vi "storageLow.vi"(8 "error in (no error)":errorcluster, 11 "reference in":refnum<class "Project Panels.lvclass">=refnum) -> (0 "error out":errorcluster={"status"=TRUE, "code"=1556, "source"="In Place Element Structure in Project Panels.lvclass:items.vi"}, 2 "saved?":bool, 3 "reference out":refnum<class "Project Panels.lvclass">)   [LabVIEW 2016, in "Project Panels.lvclass"]
uses:
  Project Panels.lvclass
  SYS/Items Controller_llb/storageSheets.ctl
  stateItem.ctl
  <vilib>/Utility/miscctls.llb/LVRowAndColumnUnsignedTypeDef.ctl
  <vilib>/Utility/miscctls.llb/LVRowAndColumnTypeDef.ctl
  SYS/Items Controller_llb/Items Controller.lvclass
  SYS/File Controller_llb/File Controller.lvclass
panel:
  out "title":string="Cosmed Asia Pacific - Storage"
  in  "tables":enum32{"Check IN", "Check OUT", "Storage"}(tab)
  in  "checkIN":string[][](table)
  in  "checkOUT":string[][](table)
  in  "Storage":string[][](table)
  in  "uploadFile":bool
  in  "Add Check OUT":bool
  in  "Add Check IN":bool
  out "Number of Items:":i32
  out "index":i32
  in  "back":bool
  in  "next":bool
  out "storageSheets":T1
  in  "Search Item":bool
  in  "Save":bool
  out "Item Selected (S/N or P/N):":string
  out "statuBar":string="Stoped for an Error"
  in  "Stop Button":bool
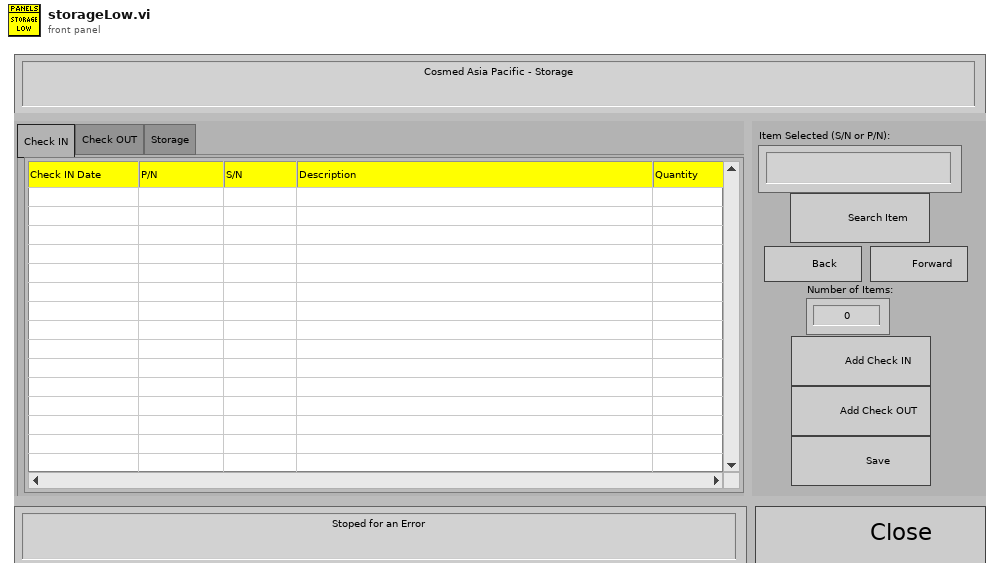
[diagram p1: front panel]
types:
  T1 = typedef "Items Controller.lvclass/storageSheets.ctl" = enum16{"check-in", "check-out", "storage"}
  T2 = typedef "Project Panels.lvclass/stateItem.ctl" = enum16{"initiate", "waitEvent", "save", "search", "UploadFile", "nextItems", "stop"}
  T3 = typedef "LVRowAndColumnUnsignedTypeDef.ctl" = cluster{"Row":u32, "Column":u32}
  T4 = enum8{"Enabled", "Disabled", "Disabled and Grayed Out"}
  T5 = cluster{"checkIN":string[][], "checkOUT":string[][], "storage":string[][]}
  T6 = typedef "LVRowAndColumnTypeDef.ctl" = cluster{"Row":i32, "Column":i32}
  T7 = typedef "Project Panels.lvclass/ObjectAttributesRef.ctl" = refnum<data-value>
  T8 = typedef "Project Panels.lvclass/ObjectAttributes.ctl" = cluster{"MyAttribute":dbl, "device_controller_ref":refnum<class "Devices Controller.lvclass">, "file_controller_ref":refnum<class "File Controller.lvclass">, "item_controller_ref":refnum<class "Items Controller.lvclass">, "item_tables":cluster{"checkIN":string[][], "checkOUT":string[][], "storage":string[][]}, "quickbook_table":cluster{"notes":string[][]}, "notification_controller_ref":refnum<class "Notification Controller.lvclass">, "partstracking_controller_ref":refnum<class "PartsTracking Controller.lvclass">, "product_tables":cluster{"k4b2":string[][], "fitmate":string[][], "RMR":string[][], "CPET":string[][], "BP":string[][], "PP":string[][], "k5":string[][], "bb-pft":string[][]}, "rowsColour":u32[], "low_resolution?":bool, "run_python?":bool}
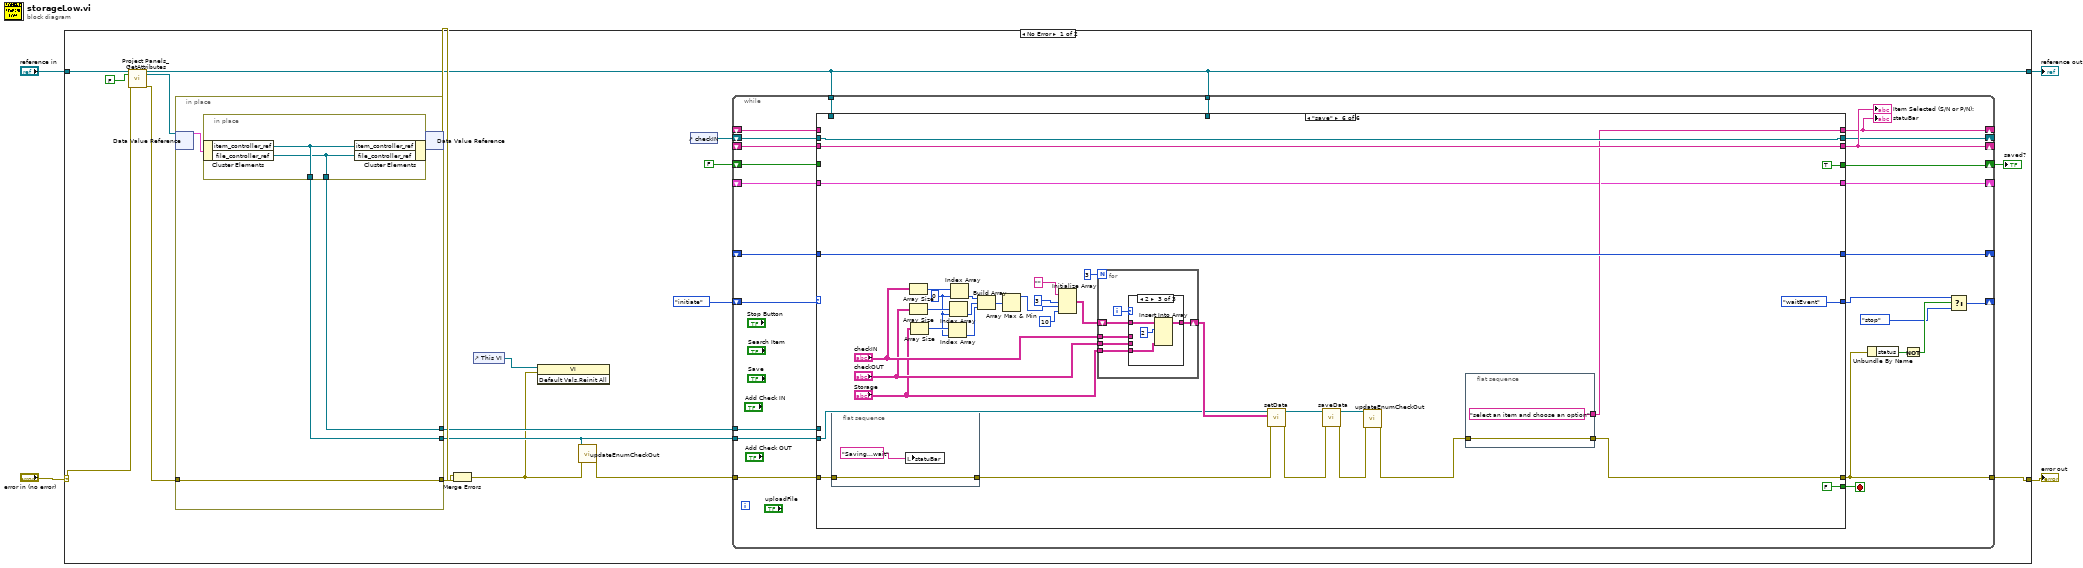
[diagram p0: block diagram]
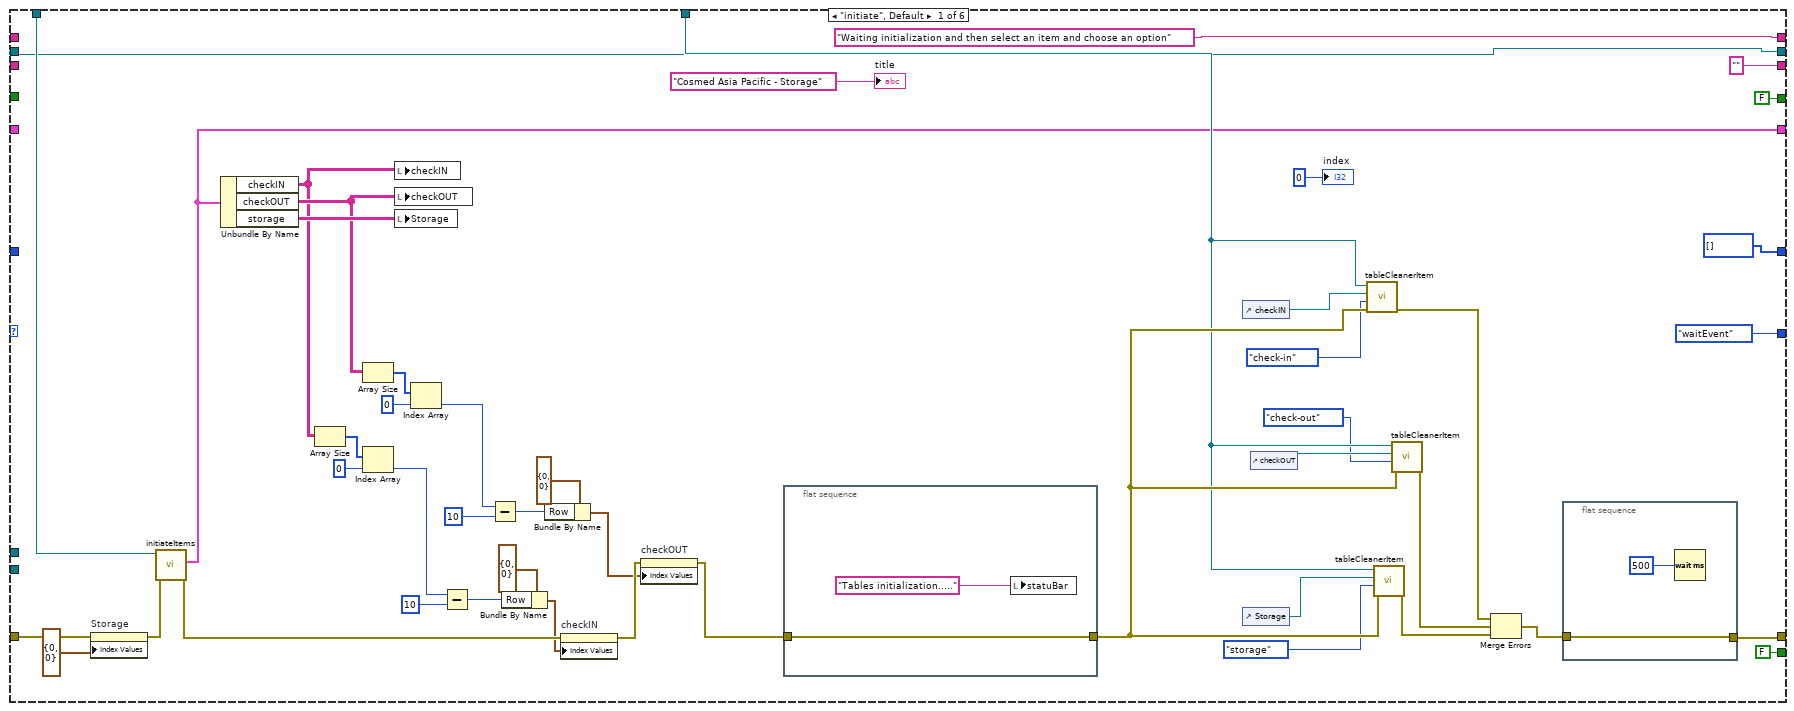
[diagram p2: hidden frame]
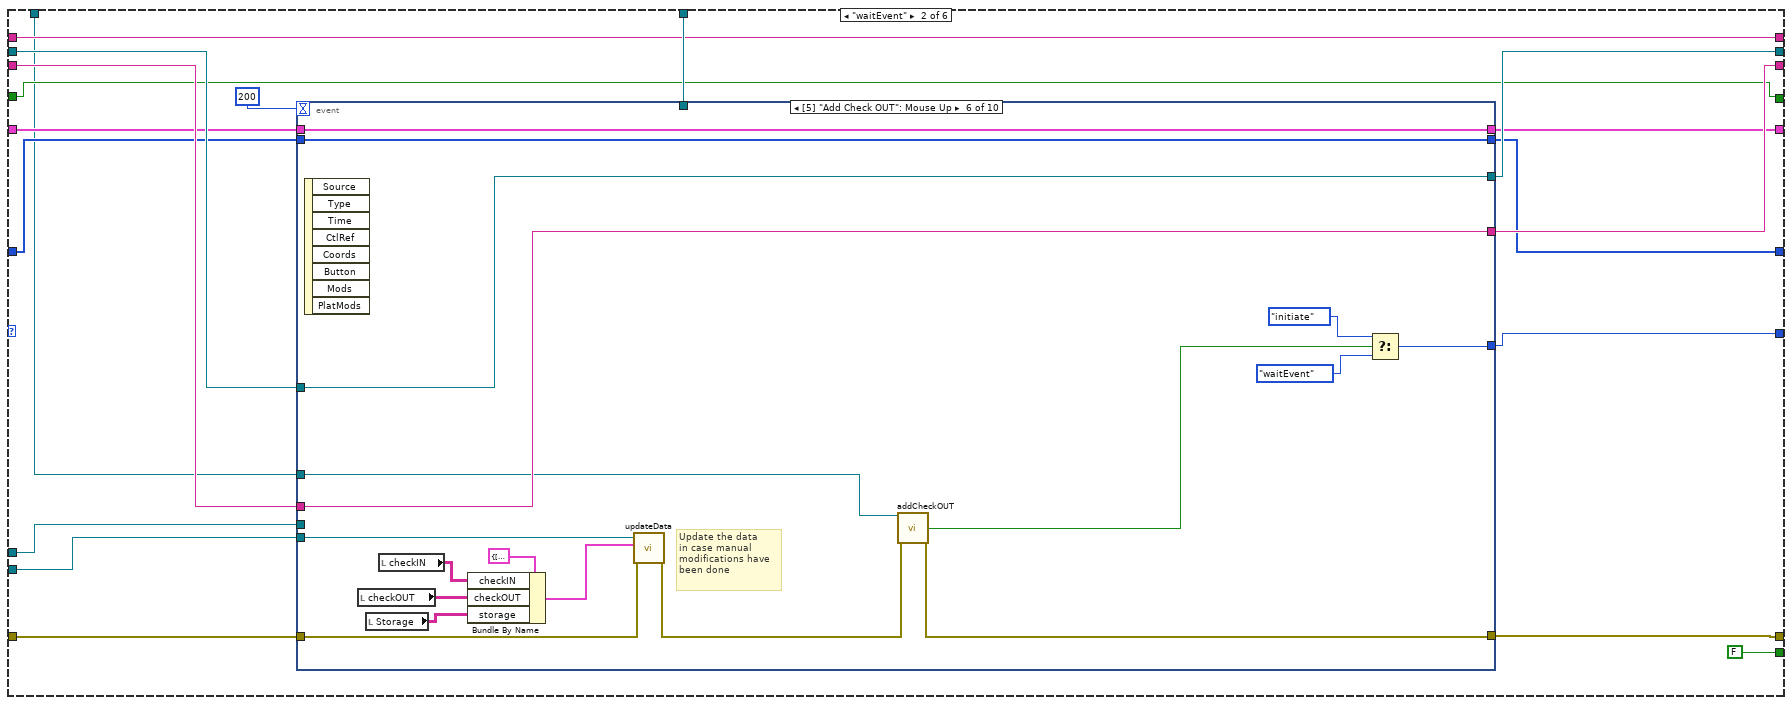
[diagram p3: hidden frame]
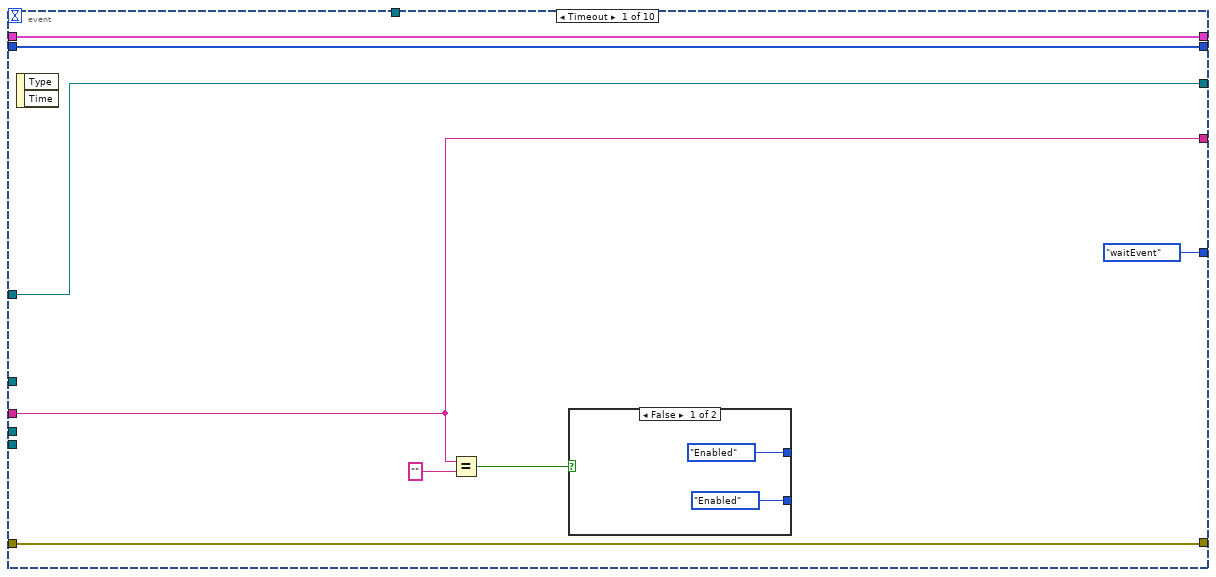
[diagram p4: hidden frame]
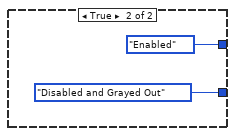
[diagram p5: hidden frame]
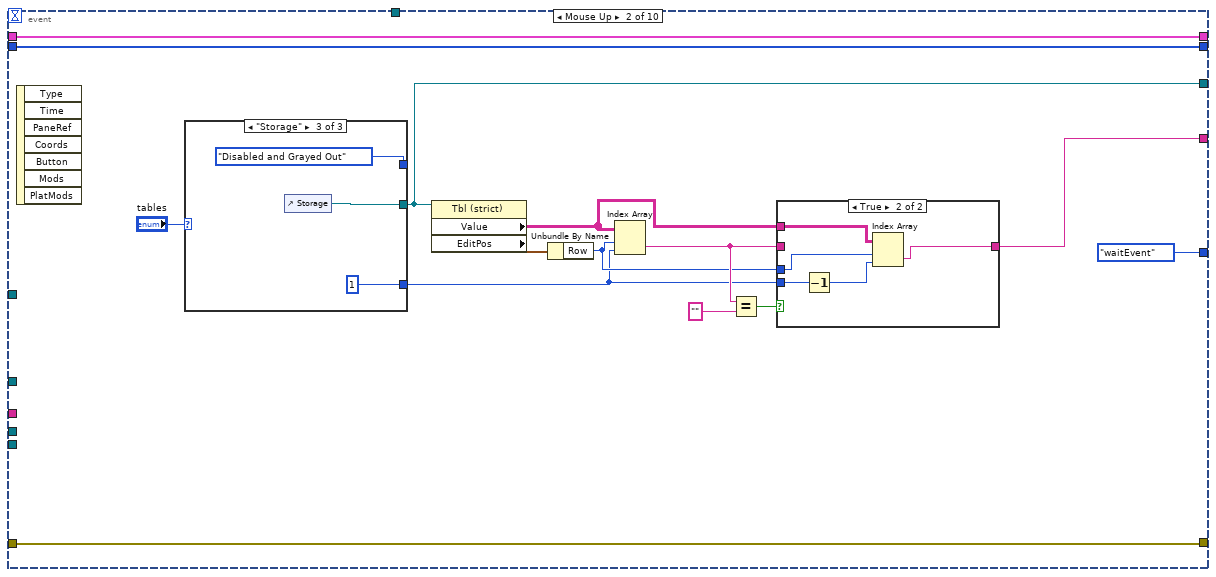
[diagram p6: hidden frame]
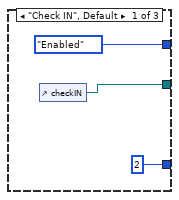
[diagram p8: hidden frame]
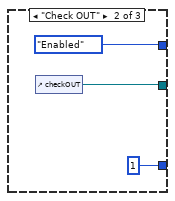
[diagram p9: hidden frame]
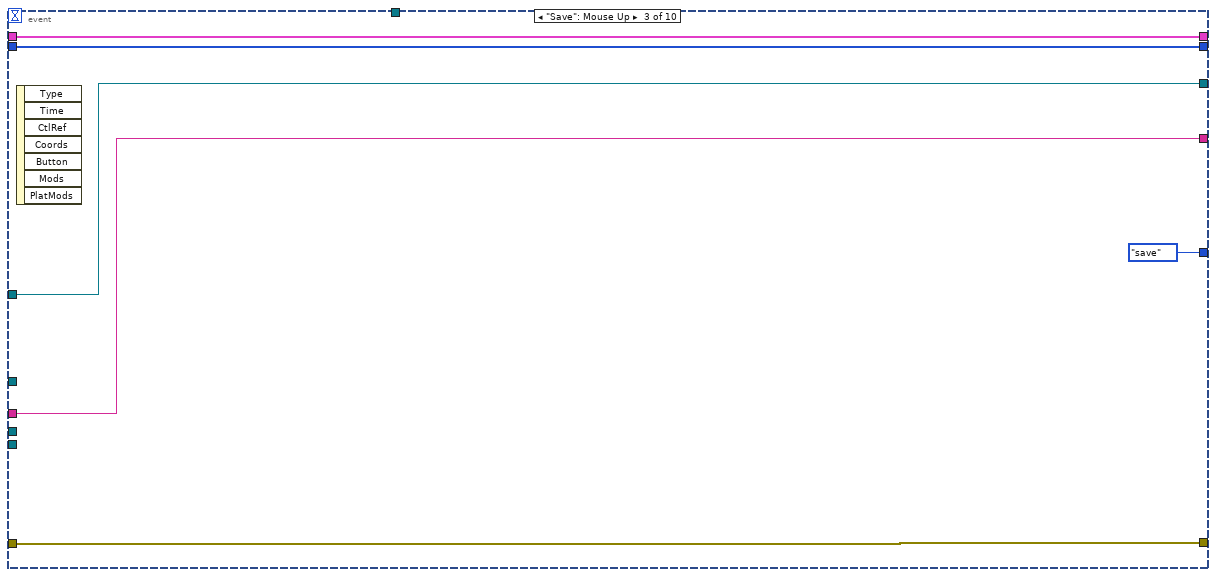
[diagram p10: hidden frame]
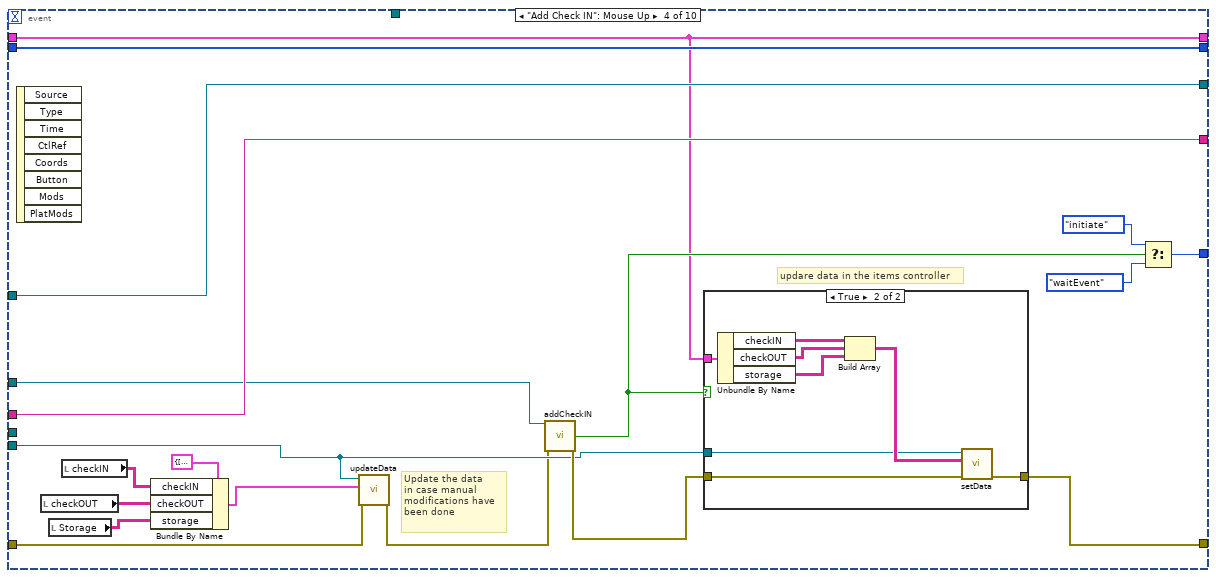
[diagram p11: hidden frame]
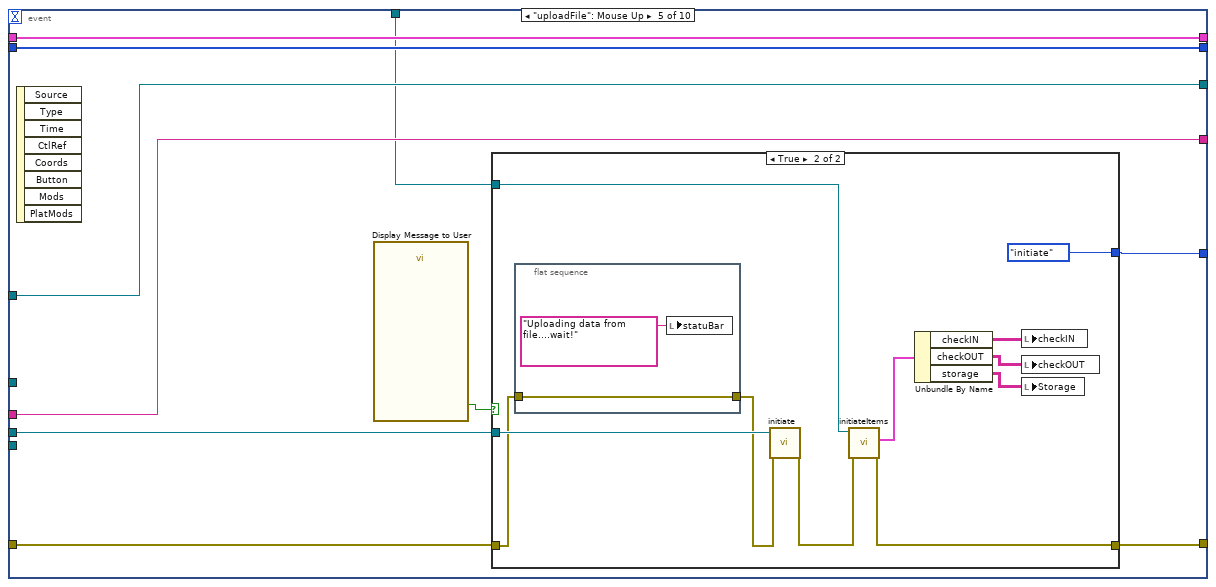
[diagram p13: hidden frame]
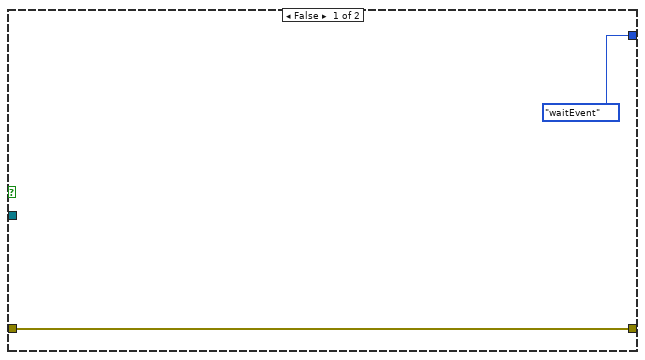
[diagram p14: hidden frame]
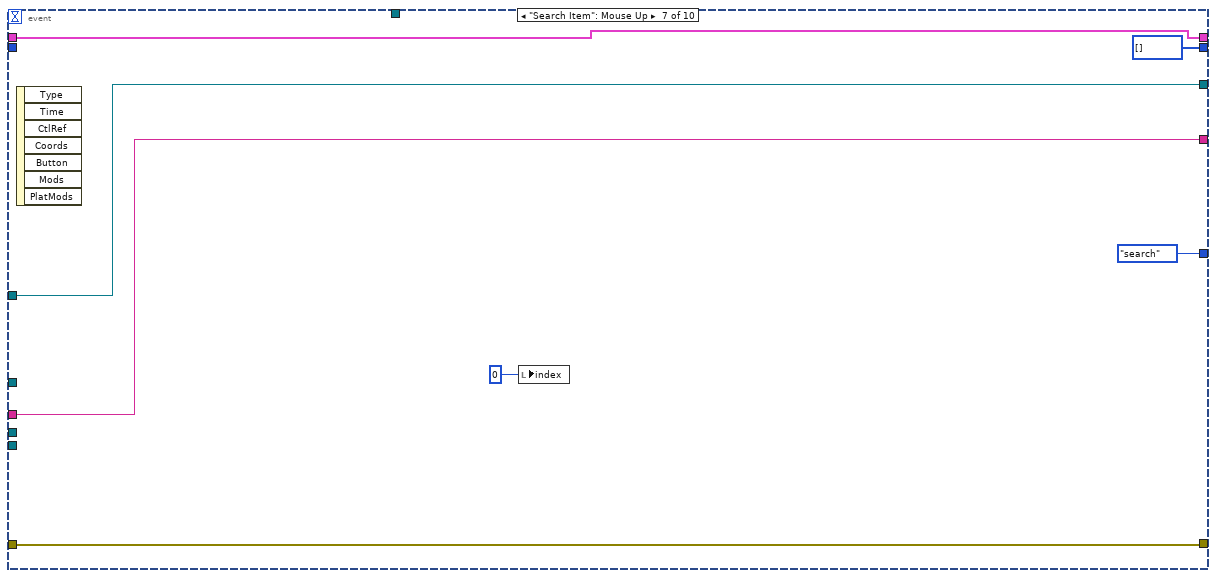
[diagram p15: hidden frame]
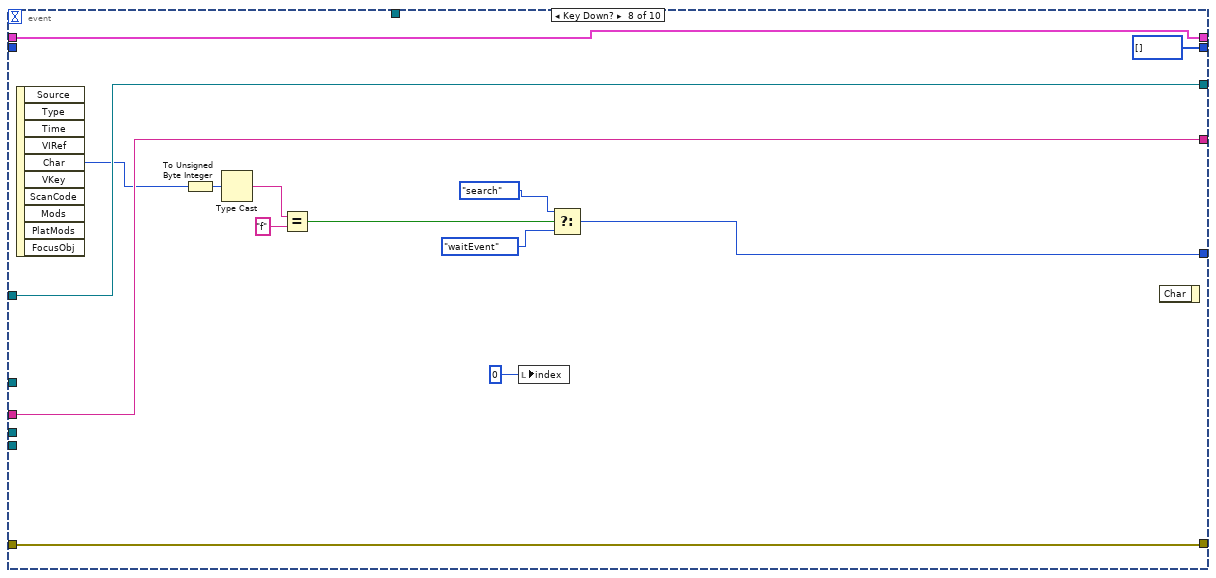
[diagram p16: hidden frame]
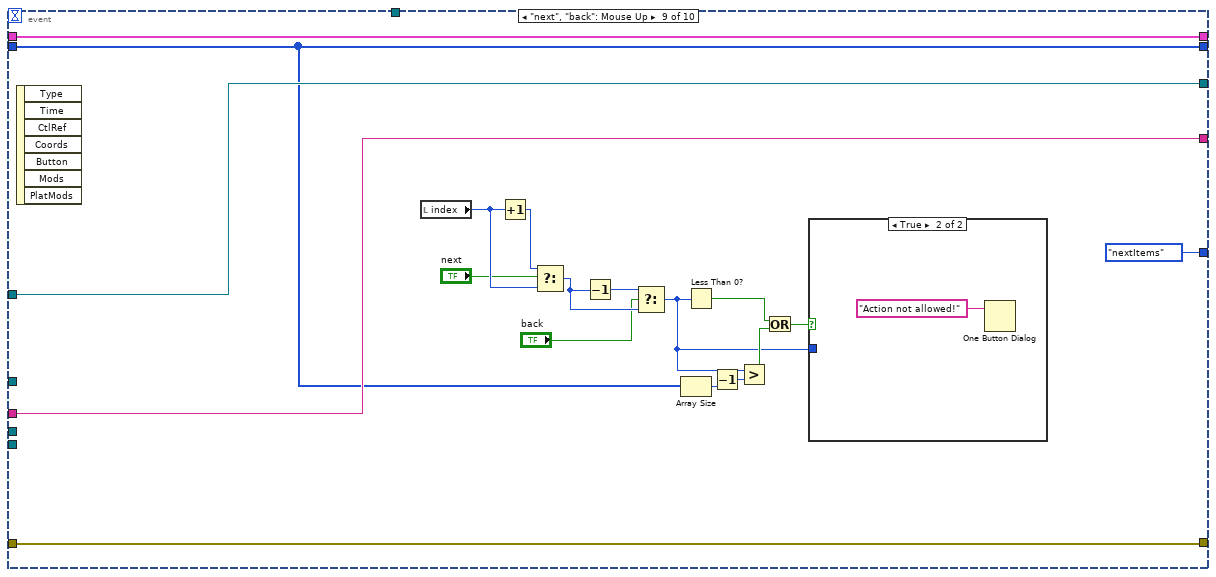
[diagram p17: hidden frame]
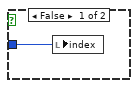
[diagram p18: hidden frame]
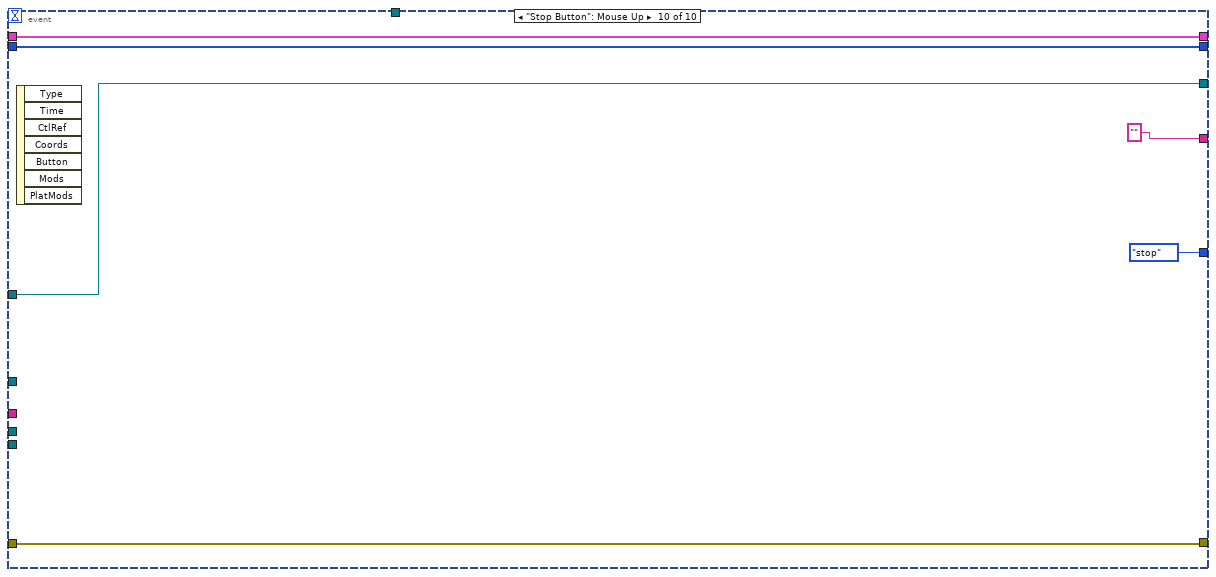
[diagram p19: hidden frame]
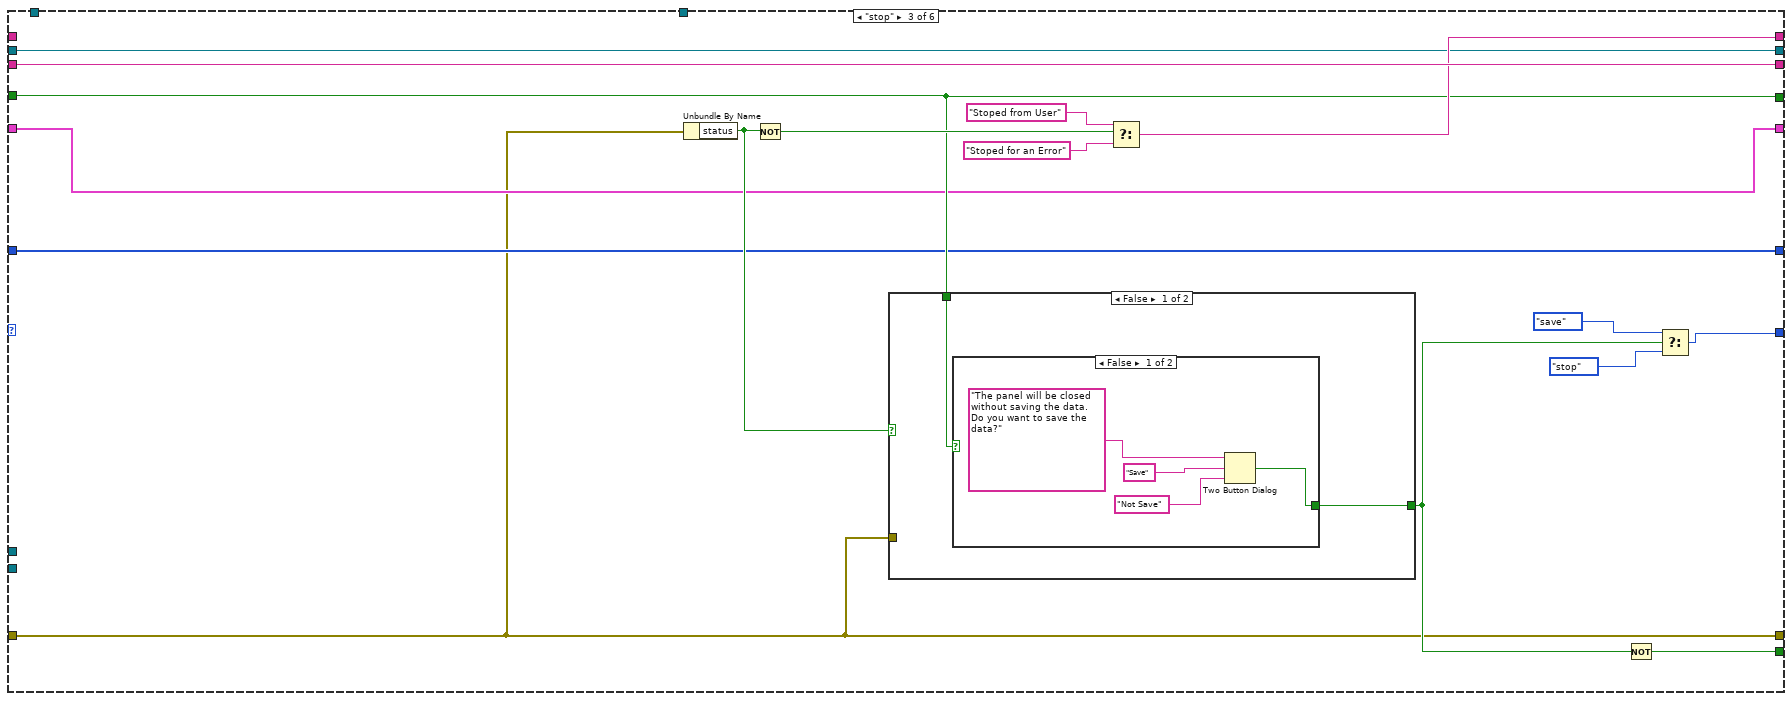
[diagram p20: hidden frame]
diagram:
  n1 = case shown="No Error" "error in (no error)" {
    selector: "error in (no error)" -> [w18 w415]
    tunnel: [w15 w415] -> w3
    tunnel: [w13 w414] -> w1
    tunnel: "reference in" -> [w20 w414]
    frame No Error {
      n2 = call "Project Panels_GetAttributes.vi"("reference in"=w20, "return data? (T)"=FALSE, "error in (no error)"=w18) -> ("reference out"=w13:refnum<class "Project Panels.lvclass">, "attributes ref"=w16:T7, "error out"=w17:errorcluster)  [unwired: 13 in, 1 out]
      n3 = in-place {
        in-place-border: w17 -> [w409]
        in-place-border: [w409] -> w21
        in-place-border: [w408] -> w7
        in-place-border: [w407] -> w8
        n4 = in-place-dvr #1(w16) -> (w410:T8)  [unwired: 1 out]
        n5 = in-place {
          in-place-border: [w413] -> w408
          in-place-border: [w412] -> w407
          n6 = in-place-cluster #2(w410) -> ("item_controller_ref"=w413:refnum<class "Items Controller.lvclass">, "file_controller_ref"=w412:refnum<class "File Controller.lvclass">)
          n7 = in-place-cluster #2("item_controller_ref"=w413, "file_controller_ref"=w412) -> (w411:T8)
        }
        n8 = in-place-dvr #1(w411) -> (w22:errorcluster)  [unwired: 1 out]
      }
      n9 = Merge Errors(w21, w22) -> (w6:errorcluster)
      n10 = control-ref of="This VI"() -> (w11:refnum<vi>)
      n11 = invoke class="VI" method="Default Vals.Reinit All"(reference=w11, error in=w6) -> ()  [unwired: 1 in, 3 out]
      n12 = call "updateEnumCheckOut.vi"("reference in"=w7, "error in (no error)"=w6) -> ("error out"=w5:errorcluster)  [unwired: 16 in, 1 out]
      n13 = control-ref of="checkIN"() -> (w12:refnum<vi>)
      n14 = while {
        tunnel: w13 -> [w47]
        tunnel: w5 -> [w46]
        tunnel: [w44] -> w15
        shift-right: [w41] -> _
        shift-left: stateItem."initiate" ("state") -> [w45]
        shift-right: [w38] -> _
        shift-left: _ -> [w37]
        shift-right: [w36] -> _
        shift-left: w12 -> [w35]
        tunnel: w13 -> [w34]
        tunnel: w7 -> [w32]
        shift-right: [w30] -> w9
        shift-left: FALSE -> [w31]
        shift-right: [w29] -> _
        shift-left: _ -> [w28]
        shift-right: [w27] -> _
        shift-left: _ -> [w26]
        shift-right: [w25] -> _
        shift-left: _ -> [w24]
        tunnel: w8 -> [w23]
        stop <- w39 stop-if-true
        n15 = case shown="\"save\"" w45 {
          tunnel: w47 -> [w82 w107 _ _ _ _]
          tunnel: w46 -> [w75 w116 w283 w311 w343 w380]
          tunnel: [w85 w110 w283 w322 w343 w377] -> w44
          tunnel: [stateItem."waitEvent" ("state") w109 w289 w317 stateItem."waitEvent" ("state") stateItem."waitEvent" ("state")] -> w42
          tunnel: [FALSE FALSE w288 FALSE FALSE FALSE] -> w39
          tunnel: ["Waiting initialization and then select an item and choose an option" ("title") w105 w295 "Search Item option selected..." ("title") "Click on the arrows to select other items" ("title") w376] -> w29
          tunnel: ["" w112 w298 w323 w340 w381] -> w38
          tunnel: w37 -> [_ w114 w298 w323 w340 w381]
          tunnel: [w79 w111 w294 w324 w334 w382] -> w36
          tunnel: w35 -> [w79 w113 w294 w324 w334 w382]
          tunnel: w34 -> [w81 w100 _ w313 _ _]
          tunnel: w32 -> [_ w108 _ _ _ w354]
          tunnel: w31 -> [_ w106 w287 w321 w341 _]
          tunnel: [FALSE w106 w287 w321 w341 TRUE] -> w30
          tunnel: w28 -> [_ w105 _ _ _ _]
          tunnel: [i32[] [] ("indexElements") w103 w286 w315 w335 w378] -> w27
          tunnel: w26 -> [_ w104 w286 _ w335 w378]
          tunnel: [w48 w101 w285 w312 w327 w375] -> w25
          tunnel: w24 -> [_ w102 w285 w312 w327 w375]
          tunnel: w23 -> [_ w99 _ _ _ _]
          frame "initiate", Default {
            n16 = property on="Storage" class="Tbl (strict)"(error in=w75, "Index Values"=T3 {"Row"=0, "Column"=0}) -> (error out=w74:errorcluster)  [unwired: 1 in, 1 out]
            n17 = call "initiateItems.vi"("error in (no error)"=w74, "reference in"=w81) -> ("error out"=w66:errorcluster, "table"=w48:T5)  [unwired: 7 in, 1 out]
            n18 = Unbundle By Name(w48) -> ("checkIN"=w49:string[][], "checkOUT"=w68:string[][], "storage"=w73:string[][])
            n19 = Array Size(array=w49) -> (size(s)=w55:i32[])
            n20 = Array Size(array=w68) -> (size(s)=w62:i32[])
            n21 = Index Array(array=w55, index=0) -> (element=w52:i32)
            n22 = local write "checkIN"(w49) -> ()
            n23 = local write "checkOUT"(w68) -> ()
            n24 = local write "Storage"(w73) -> ()
            n25 = Index Array(array=w62, index=0) -> (element=w59:i32)
            n26 = Subtract(x=w52, y=10) -> (x-y=w53:i32)
            n27 = Subtract(x=w59, y=10) -> (x-y=w60:i32)
            n28 = Bundle By Name(cluster=T3 {"Row"=0, "Column"=0} ("Index Values"), "Row"=w53) -> (w50:T3)
            n29 = Bundle By Name(cluster=T3 {"Row"=0, "Column"=0} ("Index Values"), "Row"=w60) -> (w57:T3)
            n30 = property on="checkIN" class="Tbl (strict)"(error in=w66, "Index Values"=w50) -> (error out=w65:errorcluster)  [unwired: 1 in, 1 out]
            n31 = property on="checkOUT" class="Tbl (strict)"(error in=w65, "Index Values"=w57) -> (error out=w67:errorcluster)  [unwired: 1 in, 1 out]
            n32 = flat-sequence {
              tunnel: w67 -> [w96]
              tunnel: [w96] -> w84
              frame #0 {
                n33 = local write "statuBar"("Tables initialization....." ("title")) -> ()
              }
            }
            n34 = control-ref of="checkIN"() -> (w92:refnum<vi>)
            n35 = control-ref of="Storage"() -> (w94:refnum<vi>)
            n36 = control-ref of="checkOUT"() -> (w93:refnum<vi>)
            n37 = call "tableCleanerItem.vi"("error in (no error)"=w84, "storageSheets"=storageSheets."check-in", "Table in"=w92, "reference in"=w82) -> ("error out"=w91:errorcluster)  [unwired: 6 in, 1 out]
            n38 = call "tableCleanerItem.vi"("error in (no error)"=w84, "storageSheets"=storageSheets."storage", "Table in"=w94, "reference in"=w82) -> ("error out"=w89:errorcluster)  [unwired: 6 in, 1 out]
            n39 = call "tableCleanerItem.vi"("error in (no error)"=w84, "storageSheets"=storageSheets."check-out", "Table in"=w93, "reference in"=w82) -> ("error out"=w90:errorcluster)  [unwired: 6 in, 1 out]
            n40 = Merge Errors(w91, w90, w89) -> (w80:errorcluster)
            n41 = flat-sequence {
              tunnel: w80 -> [w98]
              tunnel: [w98] -> w85
              frame #0 {
                n42 = Wait (ms)(milliseconds to wait=u32 500) -> ()  [unwired: 1 out]
              }
            }
            "title" <- "Cosmed Asia Pacific - Storage" ("title")
            "index" <- 0 ("index")
          }
          frame "waitEvent" {
            n43 = event shown="[5] \"Add Check OUT\": Mouse Up" {
              selector: _ -> [_ _ _ _ _ _ _ _ _ _]
              dyn-events: _ -> [_ _ _ _ _ _ _ _ _ _]
              timeout: 200 -> [_ _ _ _ _ _ _ _ _ _]
              tunnel: w116 -> [w125 w143 w159 w171 w198 w226 w239 w254 w274 w282]
              tunnel: [w125 w143 w159 w174 w197 w231 w239 w254 w274 w282] -> w110
              tunnel: w114 -> [w121 _ w163 w183 w199 w235 w241 w255 w267 _]
              tunnel: w113 -> [w122 _ w164 w182 w200 w234 w242 w256 w268 w280]
              tunnel: [w121 w136 w163 w183 w199 w235 w241 w255 w267 ""] -> w112
              tunnel: [w122 w140 w164 w182 w200 w234 w242 w256 w268 w280] -> w111
              tunnel: [stateItem."waitEvent" ("state") stateItem."waitEvent" ("state") stateItem."save" ("state") w178 w195 w229 stateItem."search" ("state") w244 stateItem."nextItems" ("state") stateItem."stop" ("state")] -> w109
              tunnel: w108 -> [_ _ _ w173 _ w224 _ _ _ _]
              tunnel: w107 -> [_ _ _ _ w193 _ _ _ _ _]
              tunnel: w104 -> [w119 w131 w161 w181 w201 w233 _ _ w266 w278]
              tunnel: [w119 w131 w161 w181 w201 w233 i32[] [] ("indexElements") i32[] [] ("indexElements") w266 w278] -> w103
              tunnel: w102 -> [w118 w130 w160 w172 w202 w223 w236 w251 w257 w277]
              tunnel: [w118 w130 w160 w172 w202 w223 w236 w251 w257 w277] -> w101
              tunnel: w100 -> [_ _ _ w180 _ w232 _ _ _ _]
              tunnel: w99 -> [_ _ _ _ w194 _ _ _ _ _]
              event Timeout {
                n44 = event-data() -> ()  [unwired: 1 in, 2 out]
                n45 = Equal?(x=w121, y="") -> (x = y?=w124:bool)
                n46 = case shown="False" w124 {
                  tunnel: [T4."Enabled" ("Disabled") T4."Disabled and Grayed Out" ("Disabled")] -> _
                  tunnel: [T4."Enabled" ("Disabled") T4."Enabled" ("Disabled")] -> _
                  frame False {
                  }
                  frame True {
                  }
                }
              }
              event Mouse Up {
                n47 = event-data() -> ()  [unwired: 1 in, 7 out]
                n48 = case shown="\"Storage\"" "tables" {
                  tunnel: [w152 w155 w158] -> w140
                  tunnel: [T4."Enabled" ("Disabled") T4."Enabled" ("Disabled") T4."Disabled and Grayed Out" ("Disabled")] -> _
                  tunnel: [2 ("disabled index (col)") 1 ("disabled index (col)") 1 ("disabled index (col)")] -> w133
                  frame "Check IN", Default {
                    n49 = control-ref of="checkIN"() -> (w152:refnum<vi>)
                  }
                  frame "Check OUT" {
                    n50 = control-ref of="checkOUT"() -> (w155:refnum<vi>)
                  }
                  frame "Storage" {
                    n51 = control-ref of="Storage"() -> (w158:refnum<vi>)
                  }
                }
                n52 = property on="Property Node" class="Tbl (strict)"(reference=w140) -> ("Value"=w135:string[][], "EditPos"=w142:T6)  [unwired: 1 in, 2 out]
                n53 = Unbundle By Name(w142) -> ("Row"=w134:i32)
                n54 = Index Array(array=w135, index (row)=w134, index (col)=w133) -> (element=w137:string)
                n55 = Equal?(x=w137, y="") -> (x = y?=w138:bool)
                n56 = case shown="True" w138 {
                  tunnel: w137 -> [w144 _]
                  tunnel: [w144 w145] -> w136
                  tunnel: w135 -> [_ w149]
                  tunnel: w134 -> [_ w148]
                  tunnel: w133 -> [_ w147]
                  frame False {
                  }
                  frame True {
                    n57 = Decrement(x=w147) -> (x-1=w146:i32)
                    n58 = Index Array(array=w149, index (row)=w148, index (col)=w146) -> (element=w145:string)
                  }
                }
              }
              event "Save": Mouse Up {
                n59 = event-data() -> ()  [unwired: 1 in, 7 out]
              }
              event "Add Check IN": Mouse Up {
                # "Update the data\nin case manual\nmodifications have\nbeen done"
                # "updare data in the items controller"
                n60 = event-data() -> ()  [unwired: 1 in, 8 out]
                n61 = local read "checkOUT"() -> (w167:string[][])
                n62 = local read "Storage"() -> (w166:string[][])
                n63 = local read "checkIN"() -> (w168:string[][])
                n64 = Bundle By Name(cluster=T5 {"checkIN"=[], "checkOUT"=[], "storage"=[]} ("table"), "checkIN"=w168, "checkOUT"=w167, "storage"=w166) -> (w165:T5)
                n65 = call "updateData.vi"("error in (no error)"=w171, "table"=w165, "reference in"=w173) -> ("error out"=w170:errorcluster)  [unwired: 7 in, 1 out]
                n66 = call "addCheckIN.vi"("reference in"=w180, "error in (no error)"=w170) -> ("saved?"=w176:bool, "error out"=w175:errorcluster)  [unwired: 11 in, 1 out]
                n67 = case shown="True" w176 {
                  tunnel: w172 -> [_ w188]
                  tunnel: w175 -> [w184 w187]
                  tunnel: [w184 w186] -> w174
                  tunnel: w173 -> [_ w185]
                  frame False {
                  }
                  frame True {
                    n68 = Unbundle By Name(w188) -> ("checkIN"=w192:string[][], "checkOUT"=w191:string[][], "storage"=w190:string[][])
                    n69 = Build Array(w192, w191, w190) -> (w189:string[][][])
                    n70 = call "setData.vi"("error in (no error)"=w187, "data"=w189, "reference in"=w185) -> ("error out"=w186:errorcluster)  [unwired: 7 in, 1 out]
                  }
                }
                n71 = Select(t=stateItem."initiate" ("state"), s=w176, f=stateItem."waitEvent") -> (s? t:f=w178:T2)
              }
              event "uploadFile": Mouse Up {
                n72 = event-data() -> ()  [unwired: 1 in, 8 out]
                n73 = call "Display Message to User"() -> ("Yes"=w196:bool)  [unwired: 10 in, 1 out]
                n74 = case shown="True" w196 {
                  tunnel: w198 -> [w204 w206]
                  tunnel: [w204 w210] -> w197
                  tunnel: [stateItem."waitEvent" ("state") stateItem."initiate" ("state")] -> w195
                  tunnel: w194 -> [_ w214]
                  tunnel: w193 -> [_ w212]
                  frame False {
                  }
                  frame True {
                    n75 = flat-sequence {
                      tunnel: w206 -> [w217]
                      tunnel: [w217] -> w205
                      frame #0 {
                        n76 = local write "statuBar"("Uploading data from file....wait!" ("statuBar")) -> ()
                      }
                    }
                    n77 = call "initiate.vi"("reference in"=w214, "error in (no error)"=w205) -> ("error out"=w211:errorcluster)  [unwired: 16 in, 1 out]
                    n78 = call "initiateItems.vi"("error in (no error)"=w211, "reference in"=w212) -> ("error out"=w210:errorcluster, "table"=w213:T5)  [unwired: 7 in, 1 out]
                    n79 = Unbundle By Name(w213) -> ("checkIN"=w209:string[][], "checkOUT"=w208:string[][], "storage"=w207:string[][])
                    n80 = local write "checkIN"(w209) -> ()
                    n81 = local write "checkOUT"(w208) -> ()
                    n82 = local write "Storage"(w207) -> ()
                  }
                }
              }
              event "Add Check OUT": Mouse Up {
                # "Update the data\nin case manual\nmodifications have\nbeen done"
                n83 = event-data() -> ()  [unwired: 1 in, 8 out]
                n84 = local read "checkOUT"() -> (w220:string[][])
                n85 = local read "Storage"() -> (w219:string[][])
                n86 = local read "checkIN"() -> (w221:string[][])
                n87 = Bundle By Name(cluster=T5 {"checkIN"=[], "checkOUT"=[], "storage"=[]} ("table"), "checkIN"=w221, "checkOUT"=w220, "storage"=w219) -> (w218:T5)
                n88 = call "updateData.vi"("error in (no error)"=w226, "table"=w218, "reference in"=w224) -> ("error out"=w225:errorcluster)  [unwired: 7 in, 1 out]
                n89 = call "addCheckOUT.vi"("reference in"=w232, "error in (no error)"=w225) -> ("saved?"=w228:bool, "error out"=w231:errorcluster)  [unwired: 11 in, 1 out]
                n90 = Select(t=stateItem."initiate" ("state"), s=w228, f=stateItem."waitEvent") -> (s? t:f=w229:T2)
              }
              event "Search Item": Mouse Up {
                n91 = event-data() -> ()  [unwired: 1 in, 7 out]
                n92 = local write "index"(0 ("index")) -> ()
              }
              event Key Down? {
                n93 = event-data() -> ("Char"=w249:i16)  [unwired: 1 in, 9 out]
                n94 = To Unsigned Byte Integer(number=w249) -> (unsigned 8bit integer=w250:u8)
                n95 = Type Cast(x=w250) -> (*(type *) &x=w248:string)  [unwired: 1 in]
                n96 = Equal?(x=w248, y="f") -> (x = y?=w243:bool)
                n97 = local write "index"(0 ("index")) -> ()
                n98 = Select(t=stateItem."search" ("state"), s=w243, f=stateItem."waitEvent" ("state")) -> (s? t:f=w244:T2)
                n99 = event-data() -> ()  [unwired: 2 in, 1 out]
              }
              event "next", "back": Mouse Up {
                n100 = event-data() -> ()  [unwired: 1 in, 7 out]
                n101 = local read "index"() -> (w272:i32)
                n102 = Increment(x=w272) -> (x+1=w273:i32)
                n103 = Select(t=w273, s="next", f=w272) -> (s? t:f=w270:i32)
                n104 = Decrement(x=w270) -> (x-1=w271:i32)
                n105 = Select(t=w271, s="back", f=w270) -> (s? t:f=w261:i32)
                n106 = Array Size(array=w266) -> (size(s)=w265:i32)
                n107 = Less Than 0?(x=w261) -> (x < 0?=w263:bool)
                n108 = Decrement(x=w265) -> (x-1=w258:i32)
                n109 = Greater?(x=w261, y=w258) -> (0:w264:bool)
                n110 = Or(x=w263, y=w264) -> (x .or. y?=w262:bool)
                n111 = case shown="True" w262 {
                  tunnel: w261 -> [w275 _]
                  frame False {
                    n112 = local write "index"(w275) -> ()
                  }
                  frame True {
                    n113 = One Button Dialog(message="Action not allowed!") -> ()  [unwired: 1 in, 1 out]
                  }
                }
              }
              event "Stop Button": Mouse Up {
                n114 = event-data() -> ()  [unwired: 1 in, 7 out]
              }
            }
          }
          frame "stop" {
            n115 = Unbundle By Name(w283) -> ("status"=w293:bool)
            n116 = Not(x=w293) -> (.not. x?=w292:bool)
            n117 = case shown="False" w293 {
              tunnel: w283 -> [_ w308]
              tunnel: [w300 FALSE ("Save")] -> w284
              tunnel: w287 -> [w299 _]
              frame False {
                n118 = case shown="False" w299 {
                  tunnel: [w303 FALSE ("Save")] -> w300
                  frame False {
                    n119 = Two Button Dialog(message="The panel will be closed without saving the data. Do you want to save the data?", 1:"Not Save" ("F button name (\"Cancel\")"), 2:"Save" ("T button name (\"OK\")")) -> (T button?=w303:bool)
                  }
                  frame True {
                  }
                }
              }
              frame True {
                n120 = Unbundle By Name(w308) -> ("source"=w307:string)
                n121 = Concatenate Strings("An Error occur: " ("message"), w307) -> (w310:string)
                n122 = One Button Dialog(message=w310) -> ()  [unwired: 1 in, 1 out]
              }
            }
            n123 = Select(t="Stoped from User" ("title"), s=w292, f="Stoped for an Error" ("title")) -> (s? t:f=w295:string)
            n124 = Not(x=w284) -> (.not. x?=w288:bool)
            n125 = Select(t=stateItem."save", s=w284, f=stateItem."stop" ("state")) -> (s? t:f=w289:T2)
          }
          frame "search" {
            n126 = call "searchItem.vi"("reference in"=w313, "error in (no error)"=w311) -> ("Sheet out"=→"storageSheets":T1, "indexElements"=w315:i32[], "error out"=w322:errorcluster)  [unwired: 10 in, 1 out]
            n127 = Array Size(array=w315) -> (size(s)=w314:i32)
            "Number of Items:" <- w314
            n128 = Greater Than 0?(x=w314) -> (x > 0?=w316:bool)
            n129 = Select(t=stateItem."nextItems" ("state"), s=w316, f=stateItem."waitEvent" ("state")) -> (s? t:f=w317:T2)
          }
          frame "nextItems" {
            n130 = local read "storageSheets"() -> (w330:T1)
            n131 = local read "index"() -> (w337:i32)
            n132 = case shown="\"storage\"" w330 {
              tunnel: [w345 w347 w349] -> w329
              tunnel: [enum32{"Check IN", "Check OUT", "Storage"}."Check IN" ("tables") enum32{"Check IN", "Check OUT", "Storage"}."Check OUT" ("tables") enum32{"Check IN", "Check OUT", "Storage"}."Storage" ("tables")] -> w328
              frame "check-in", Default {
                n133 = control-ref of="checkIN"() -> (w345:refnum<vi>)
              }
              frame "check-out" {
                n134 = control-ref of="checkOUT"() -> (w347:refnum<vi>)
              }
              frame "storage" {
                n135 = control-ref of="Storage"() -> (w349:refnum<vi>)
              }
            }
            n136 = Index Array(array=w335, index=w337) -> (element=w336:i32)
            n137 = Bundle By Name(cluster=T6 {"Row"=0, "Column"=0} ("Active Cell:Active Cell"), "Row"=w336, "Column"=0) -> (w331:T6)
            n138 = local write "tables"(w328) -> ()
            n139 = property on="Property Node" class="Tbl (strict)"(reference=w329, "Index Values"=w331) -> ()  [unwired: 1 in, 2 out]
          }
          frame "save" {
            w366 = 0 ("index")
            n140 = flat-sequence {
              tunnel: w380 -> [w406]
              tunnel: [w406] -> w356
              frame #0 {
                n141 = local write "statuBar"("Saving...wait" ("title")) -> ()
              }
            }
            n142 = Array Size(array="checkIN") -> (size(s)=w369:i32[])
            n143 = Array Size(array="checkOUT") -> (size(s)=w368:i32[])
            n144 = Array Size(array="Storage") -> (size(s)=w367:i32[])
            n145 = Index Array(array=w367, index=w366) -> (element=w363:i32)
            n146 = Index Array(array=w368, index=w366) -> (element=w364:i32)
            n147 = Index Array(array=w369, index=w366) -> (element=w365:i32)
            n148 = Build Array(w365, w364, w363) -> (w362:i32[])
            n149 = Array Max & Min(array=w362) -> (max value=w359:i32)  [unwired: 3 out]
            n150 = Initialize Array("", 3 ("dimension size"), w359, 10 ("dimension size")) -> (w357:string[][][])
            n151 = for {
              N: 3 -> [_]
              shift-right: [w387] -> w373
              shift-left: w357 -> [w389]
              tunnel: "checkIN" -> [w388]
              tunnel: "checkOUT" -> [w386]
              tunnel: "Storage" -> [w385]
              i -> [w390]
              n152 = case shown="2" w390 {
                tunnel: w389 -> [w394 w398 w402]
                tunnel: w388 -> [w391 _ _]
                tunnel: [w393 w397 w401] -> w387
                tunnel: w386 -> [_ w395 _]
                tunnel: w385 -> [_ _ w399]
                frame 0, Default {
                  n153 = Insert Into Array(array=w394, index (dim 0)=0 ("index (page)"), new element=w391) -> (w393:string[][][])  [unwired: 2 in]
                }
                frame 1 {
                  n154 = Insert Into Array(array=w398, index (dim 0)=1 ("disabled index (page)"), new element=w395) -> (w397:string[][][])  [unwired: 2 in]
                }
                frame 2 {
                  n155 = Insert Into Array(array=w402, index (dim 0)=2 ("disabled index (page)"), new element=w399) -> (w401:string[][][])  [unwired: 2 in]
                }
              }
            }
            n156 = call "setData.vi"("error in (no error)"=w356, "data"=w373, "reference in"=w354) -> ("error out"=w355:errorcluster, "reference out"=w353:refnum<class "Items Controller.lvclass">)  [unwired: 7 in]
            n157 = call "saveData.vi"("error in (no error)"=w355, "reference in"=w353) -> ("error out"=w351:errorcluster, "reference out"=w352:refnum<class "Items Controller.lvclass">)  [unwired: 8 in]
            n158 = call "updateEnumCheckOut.vi"("reference in"=w352, "error in (no error)"=w351) -> ("error out"=w350:errorcluster)  [unwired: 16 in, 1 out]
            n159 = flat-sequence {
              tunnel: w350 -> [w404]
              tunnel: [w404] -> w377
              tunnel: ["select an item and choose an option" ("title")] -> w376
              frame #0 {
              }
            }
          }
        }
        "statuBar" <- w29
        "Item Selected (S/N or P/N):" <- w38
        n160 = Unbundle By Name(w44) -> ("status"=w43:bool)
        n161 = Not(x=w43) -> (.not. x?=w40:bool)
        n162 = Select(t=w42, s=w40, f=stateItem."stop" ("state")) -> (s? t:f=w41:T2)
      }
      "saved?" <- w9
    }
    frame Error {
    }
  }
  "error out" <- w3
  "reference out" <- w1
